vi "TestEn.vi"() -> ()   [LabVIEW 2016]
panel:
  out "Tranisitions":dbl
  out "Enabled":bool
  out "Loops":dbl
  in  "Enable":bool
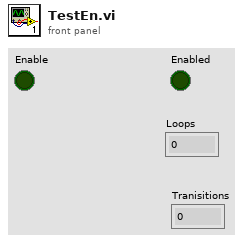
[diagram p1: front panel]
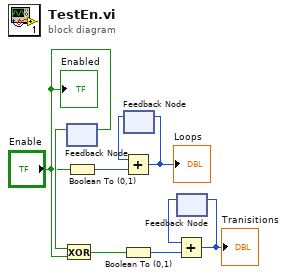
[diagram p0: block diagram]
diagram:
  n1 = feedback #1() -> (w9:bool)  [unwired: 1 in]
  n2 = Exclusive Or(1:"Enable", 2:w9) -> (0:w3:bool)
  n3 = feedback-in #1("Enable") -> ()
  n4 = Boolean To (0,1)(Boolean="Enable") -> (0, 1=w7:i16)
  n5 = Boolean To (0,1)(Boolean=w3) -> (0, 1=w4:i16)
  n6 = feedback #2() -> (w6:i16)  [unwired: 1 in]
  n7 = Add(x=w6, y=w7) -> (x+y=w5:i16)
  "Loops" <- w5
  n8 = feedback-in #2(w5) -> ()
  n9 = feedback #3() -> (w2:i16)  [unwired: 1 in]
  n10 = Add(x=w2, y=w4) -> (x+y=w1:i16)
  "Tranisitions" <- w1
  n11 = feedback-in #3(w1) -> ()
  "Enabled" <- "Enable"
